vi "Test shm put Sample arrays LV.vi"(8 "error in (no error)":errorcluster, 11 "arrays_Ctl":T1) -> (0 "error out":errorcluster, 2 "function return":i32, 3 "arrays_Ctl out":T1)   [LabVIEW 2018, in "SALLV_Test.lvlib"]
doc: "int Test_shm_putSample_arraysLV(Test_arraysLV *arrays_Ctl );"
uses:
  SALLV_Test.lvlib
  SALLV_Test.so
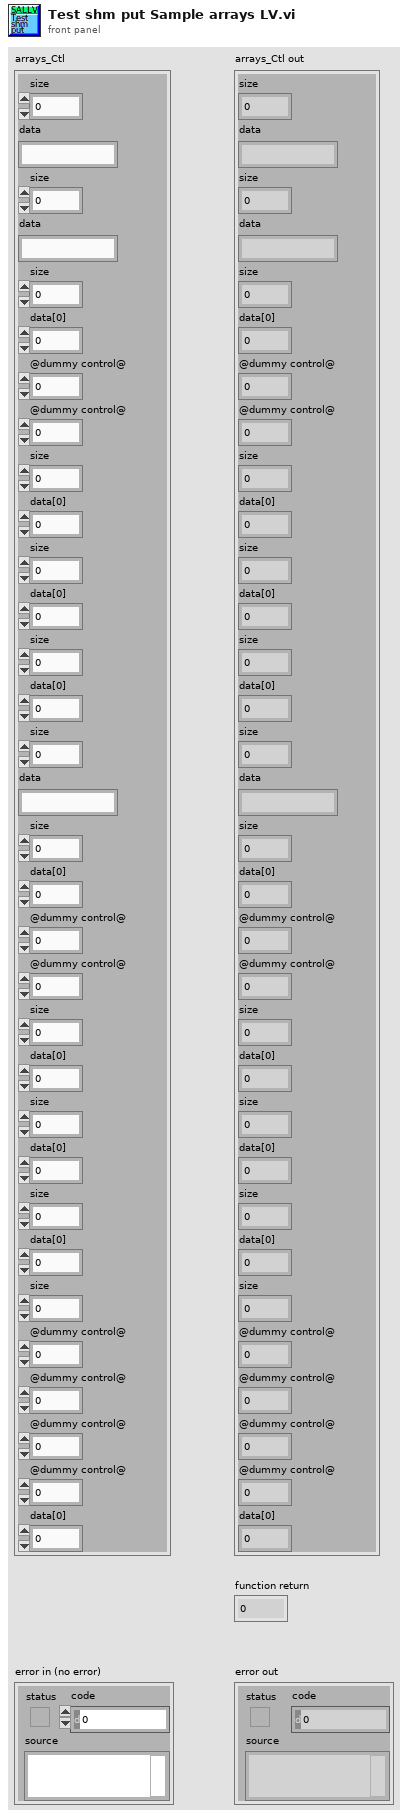
[diagram p1: front panel]
types:
  T1 = cluster{"size":i32, "data":string, "size":i32, "data":string, "size":i32, "data[0]":i16, "@dummy control@":i8, "@dummy control@":i8, "size":i32, "data[0]":i32, "size":i32, "data[0]":i32, "size":i32, "data[0]":i32, "size":i32, "data":string, "size":i32, "data[0]":u16, "@dummy control@":i8, "@dummy control@":i8, "size":i32, "data[0]":u32, "size":i32, "data[0]":u32, "size":i32, "data[0]":sgl, "size":i32, "@dummy control@":i8, "@dummy control@":i8, "@dummy control@":i8, "@dummy control@":i8, "data[0]":dbl}
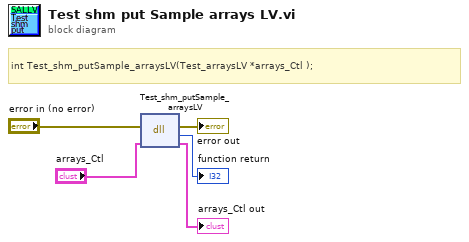
[diagram p0: block diagram]
diagram:
  # "int Test_shm_putSample_arraysLV(Test_arraysLV *arrays_Ctl );"
  n1 = dll-call lib="home/ttsai/Documents/salLabVIEWtestData/SALLV_Test.*" fn="Test_shm_putSample_arraysLV"(error in="error in (no error)", "arrays_Ctl"="arrays_Ctl") -> (error out=→"error out":errorcluster, →"function return":i32, "arrays_Ctl"=→"arrays_Ctl out":T1)  [unwired: 2 in, 1 out]
